vi "Modulo.vi"(9 "mod":dbl=2.0 format="%#_13g", 11 "input":dbl=2.0 format="%#_13g") -> (2 "round":dbl, 3 "output":dbl=2.0 format="%#_13g")   [LabVIEW 2015]
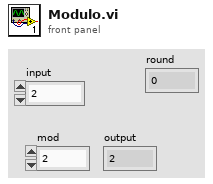
[diagram p1: front panel]
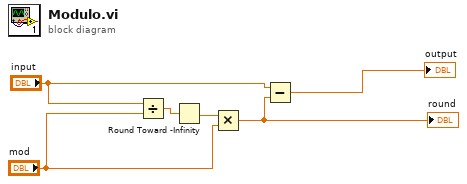
[diagram p0: block diagram]
diagram:
  n1 = Divide(x="input", y="mod") -> (x/y=w6:dbl)
  n2 = Round Toward -Infinity(1:w6) -> (0:w5:dbl)
  n3 = Multiply(x=w5, y="mod") -> (x*y=w3:dbl)
  "round" <- w3
  n4 = Subtract(x="input", y=w3) -> (x-y=→"output":dbl)
